vi "Broadcast Message.vi"(8 "error in (no error)":errorcluster, 9 "Message Data":variant, 10 "Message":string, 11 "Process In":refnum<class "Process.lvclass">) -> (0 "error out":errorcluster, 3 "Process Out":refnum<class "Process.lvclass">)   [LabVIEW 2020, in "Process.lvclass"]
doc: "Send a broadcast message to any observer who has registered for broadcast messages."
uses:
  Process.lvclass
  Broadcast Message Cluster.ctl
  Process.lvclass/Process.ctl
  Logging/Logging.lvclass
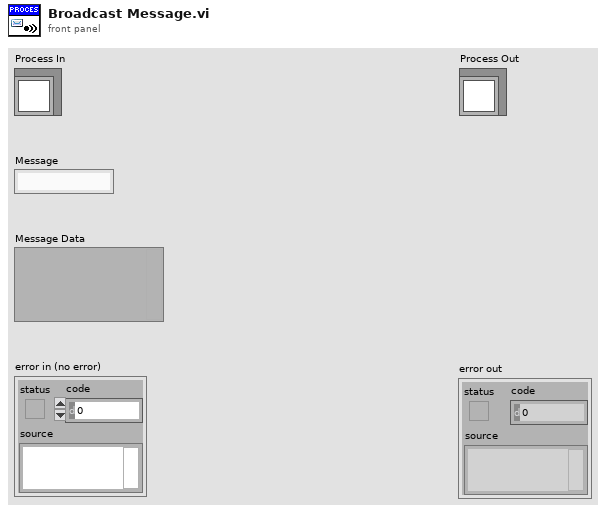
[diagram p1: front panel]
types:
  T1 = typedef "Process.lvclass/Broadcast Message Cluster.ctl" = cluster{"Sender":string, "Message":string, "Message Data":variant}
  T2 = enum16{"Send", "Receive", "Request", "Response", "Broadcast"}
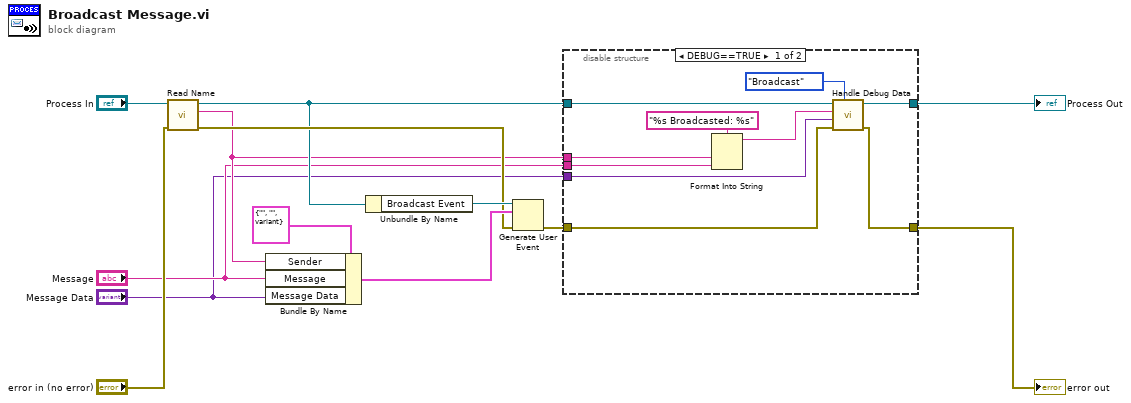
[diagram p0: block diagram]
diagram:
  n1 = call "Read Name.vi"("error in (no error)"="error in (no error)", "Process In"="Process In") -> ("error out"=w8:errorcluster, "Qualified Name"=w3:string, "Process Out"=w6:refnum<class "Process.lvclass">)  [unwired: 6 in, 1 out]
  n2 = Bundle By Name(cluster=T1 {"Sender"="", "Message"="", "Message Data"=variant} ("event data"), "Sender"=w3, "Message"="Message", "Message Data"="Message Data") -> (w10:T1)
  n3 = Unbundle By Name(w6) -> ("Broadcast Event"=w12:refnum<user-event>)
  n4 = Generate User Event(user event=w12, event data cluster=w10, error in=w8) -> (error out=w4:errorcluster)  [unwired: 1 in, 1 out]
  n5 = disable-structure shown="DEBUG==TRUE" {
    disable-tunnel: [w18 w24] -> w7
    disable-tunnel: w6 -> [w19 w25]
    disable-tunnel: [w20 w25] -> w5
    disable-tunnel: w4 -> [w17 w24]
    disable-tunnel: w3 -> [w23 _]
    disable-tunnel: "Message" -> [w22 _]
    disable-tunnel: "Message Data" -> [w15 _]
    frame condition #0 (active) {
      n6 = Format Into String(format string="%s Broadcasted: %s" ("name (unnamed)"), w23, w22) -> (resulting string=w16:string)  [unwired: 2 in, 1 out]
      n7 = call "Handle Debug Data.vi"("Action"=T2."Broadcast", "error in (no error)"=w17, "Message Data"=w15, "Message"=w16, "Process In"=w19) -> ("error out"=w18:errorcluster, "Process Out"=w20:refnum<class "Process.lvclass">)  [unwired: 5 in]
    }
    frame condition #1 {
    }
  }
  "error out" <- w7
  "Process Out" <- w5
